vi "LoadSelectedDatabase.vi"(8 "error in (no error)":errorcluster, 10 "Value":string) -> (3 "Result Set":string[][](table) caption="Result Set (from first statement with results)")   [LabVIEW 2013]
uses:
  <vilib>/drjdpowell/SQLite Library/SQL Connection/Connection.lvclass
  <vilib>/drjdpowell/SQLite Library/SQL Connection/Open (path).vi
  <vilib>/drjdpowell/SQLite Library/SQL Connection/Open (string).vi
  <vilib>/AdvancedString/Path To Command Line String.vi
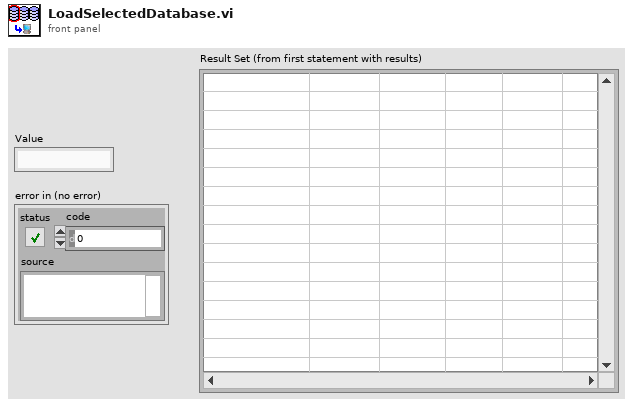
[diagram p1: front panel]
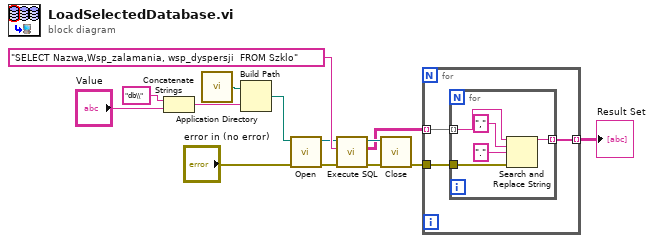
[diagram p0: block diagram]
diagram:
  n1 = Concatenate Strings("db\\" ("db file"), "Value") -> (w4:string)
  n2 = call <vilib>:"Application Directory.vi"() -> ("Application Directory"=w7:path)
  n3 = Build Path(base path=w7, name or relative path=w4) -> (appended path=w11:path)
  n4 = call-poly <vilib>:"Open.vi"("error in (no error)"="error in (no error)", "db file"=w11) -> ("error out"=w9:errorcluster, "SQLite Connection out"=w10:refnum<class "Connection.lvclass">)  [unwired: 8 in]
  n5 = call <vilib>:"Execute SQL.vi"("error in (no error)"=w9, "SQL"="SELECT Nazwa,Wsp_zalamania, wsp_dyspersji  FROM Szklo" ("SELECT  statement"), "SQLite Connection in"=w10) -> ("error out"=w6:errorcluster, "Result Set"=w3:string[][], "SQLite Connection out"=w5:refnum<class "Connection.lvclass">)  [unwired: 5 in, 1 out]
  n6 = call-dynamic "Close.vi"("error in (no error)"=w6, "SQLite Connection in"=w5) -> ("error out"=w14:errorcluster)  [unwired: 9 in]
  n7 = for {
    tunnel: w3 -> [w17] mode=indexing
    tunnel: [w16] -> w1 mode=indexing
    tunnel: w14 -> [w15]
    n8 = for {
      tunnel: w17 -> [w22] mode=indexing
      tunnel: [w19] -> w16 mode=indexing
      tunnel: w15 -> [w18]
      n9 = Search and Replace String(input string=w22, search string=",", replace string="." ("replace string (\"\")"), error in=w18) -> (result string=w19:string)  [unwired: 4 in, 3 out]
    }
  }
  "Result Set" <- w1
